vi "Temp_Set_Sub.vi"(4 "Numeric":i16, 5 "String to Write":string, 6 "NewVal":T1 format="%#_4g", 7 "Boolean":bool, 8 "error in (no error)":errorcluster, 9 "String to Write 2":string, 10 "Ring Refnum":refnum<vi>, 11 "Value":refnum<visa-resource-name>) -> (3 "dup VISA Session":refnum<visa-resource-name>)   [LabVIEW 2019]
uses:
  LS336SetTemp.ctl
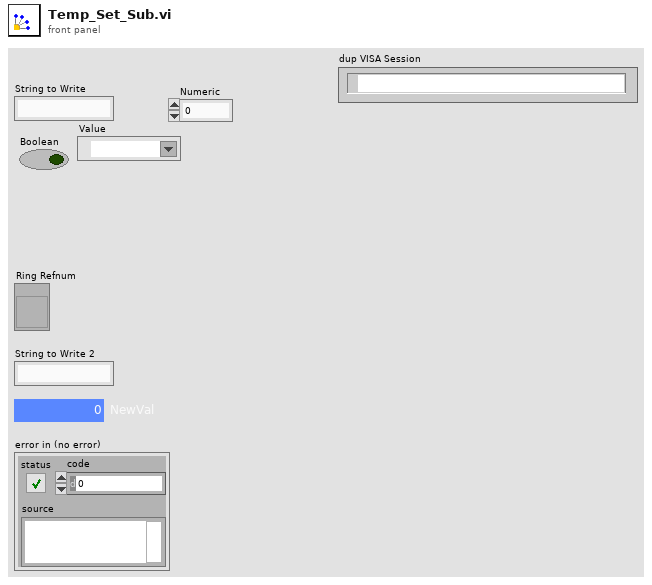
[diagram p1: front panel]
types:
  T1 = typedef "LS336SetTemp.ctl" = dbl
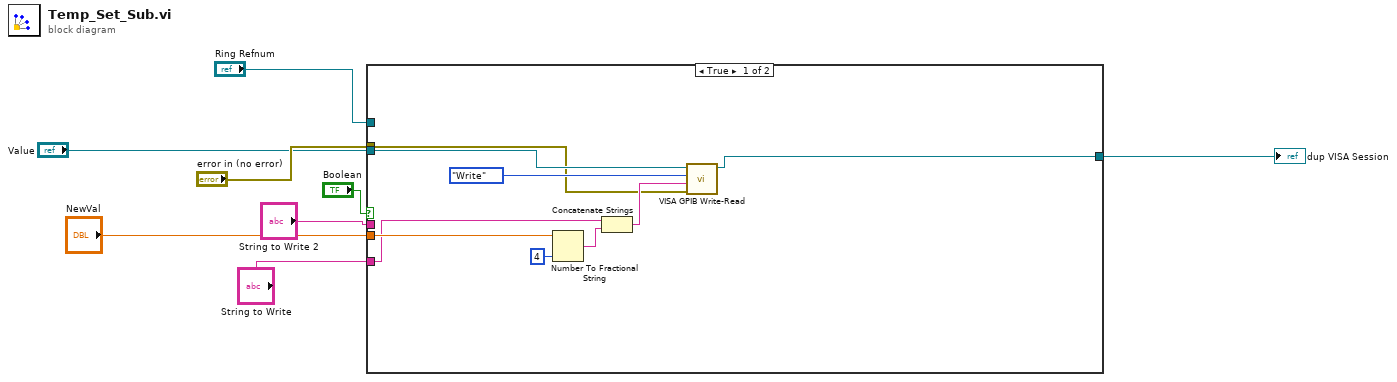
[diagram p0: block diagram]
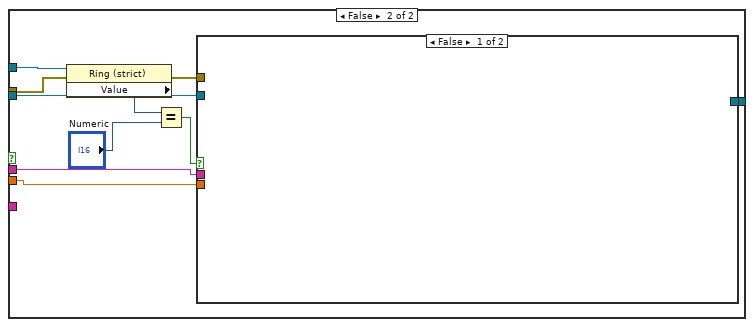
[diagram p2: hidden frame]
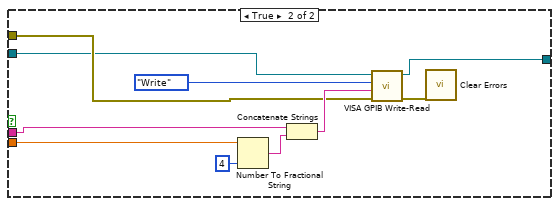
[diagram p3: hidden frame]
diagram:
  n1 = case shown="True" "Boolean" {
    tunnel: "NewVal" -> [w16 w24]
    tunnel: "error in (no error)" -> [w9 w27]
    tunnel: "String to Write 2" -> [_ w23]
    tunnel: "String to Write" -> [w12 _]
    tunnel: "Ring Refnum" -> [_ w22]
    tunnel: [w11 w20] -> w2
    tunnel: "Value" -> [w10 w18]
    frame True {
      n2 = Number To Fractional String(number=w16, precision (6)=i16 4) -> (F-format string=w14:string)  [unwired: 2 in]
      n3 = Concatenate Strings(w12, w14) -> (w13:string)
      n4 = call "VISA GPIB Write-Read.vi"("error in (no error)"=w9, "Command"=w13, "Action"=enum16{"Write", "Read", "Write & Read"}."Write", "VISA resource name"=w10) -> ("dup VISA Session"=w11:refnum<visa-resource-name>)  [unwired: 4 in, 3 out]
    }
    frame False {
      n5 = property on="Property Node" class="Ring (strict)"(reference=w22, error in=w27) -> (error out=w19:errorcluster, "Value"=w26:u16)  [unwired: 1 out]
      n6 = Equal?(x=w26, y="Numeric") -> (x = y?=w25:bool)
      n7 = case shown="False" w25 {
        tunnel: w24 -> [_ w33]
        tunnel: w23 -> [_ w31]
        tunnel: [_ w30] -> w20
        tunnel: w19 -> [_ w29]
        tunnel: w18 -> [_ w28]
        frame False {
        }
        frame True {
          n8 = Number To Fractional String(number=w33, precision (6)=i16 4) -> (F-format string=w35:string)  [unwired: 2 in]
          n9 = Concatenate Strings(w31, w35) -> (w34:string)
          n10 = call "VISA GPIB Write-Read.vi"("error in (no error)"=w29, "Command"=w34, "Action"=enum16{"Write", "Read", "Write & Read"}."Write", "VISA resource name"=w28) -> ("error out"=w32:errorcluster, "dup VISA Session"=w30:refnum<visa-resource-name>)  [unwired: 4 in, 2 out]
          n11 = call <vilib>:"Clear Errors.vi"("error in (no error)"=w32) -> ()  [unwired: 5 in, 2 out]
        }
      }
    }
  }
  "dup VISA Session" <- w2
